vi "Disable.vi"(8 "error in (no error)":errorcluster, 11 "NhRegenGridSim in":refnum<class "NHRGridSim.lvclass">) -> (0 "error out":errorcluster, 3 "NhRegenGridSim out":refnum<class "NHRGridSim.lvclass">)   [LabVIEW 2018, in "AcPwrPlugins.lvlib" / "NHRGridSim.lvclass"]
doc: "This VI turns off the unit. Off is defined as the output relay being open."
uses:
  NHRGridSim.lvclass
  <instrlib>/NH Research 9400 Series/NH Research 9400 Series.lvlib
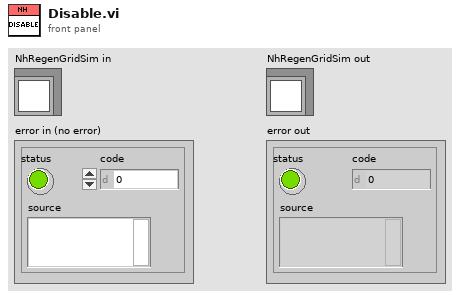
[diagram p1: front panel]
types:
  T1 = typedef "AcPwrPlugins.lvlib/NhRegenGridSim.lvclass/DeviceSettings.ctl" = cluster{"SlewRates":cluster{"Islew":dbl, "Vslew":dbl, "Pslew":dbl, "FreqSlew":dbl, "AngleABSlew":dbl, "AngleACSlew":dbl}, "Phases":cluster{"Pout (W)":dbl, "Iout (A)":dbl, "PhaseAngle":dbl, "Vout (V)":dbl, "Phase Name":string}[], "Measurement":cluster{"ApertureLength (s)":dbl, "NumberOfSamples":u32}, "Ranges":cluster{"Irange (A)":dbl, "Vrange (V)":dbl}, "Mode":enum8{"One 3-Phase AC", "One AC", "One DC", "Three AC", "Three DC", "One 2-Phase AC and One AC", "One 2-Phase AC and One DC", "Two AC", "One AC and One DC", "Two AC and One DC", "One AC and Two DC", "One DC and One AC", "Two DC"}, "PowerMax":u16, "TransformerRatio":dbl, "Waveshape":dbl[], "Handle":string, "FreqOut (Hz)":dbl, "Connected":bool, "Safety Limits":cluster{"Minimum Voltage (V)":dbl, "Minimum Voltage Time (s)":dbl, "Maximum Voltage (V)":dbl, "Maximum Voltage Time (s)":dbl, "Maximum Source Amps (A)":dbl, "Maximum Source Amps Time (s)":dbl, "Maximum Sink Amps (A)":dbl, "Maximum Sink Amps Time (s)":dbl, "Maximum Source Power (W)":dbl, "Maximum Source Power Time (s)":dbl, "Maximum Sink Power (W)":dbl, "Maximum Sink Power Time (s)":dbl, "Peak Voltage (V)":dbl, "Peak Voltage Enable":bool, "Peak Amps (A)":dbl, "Peak Amps Enable":bool}, "btnIdQuery":bool, "btnReset":bool}[]
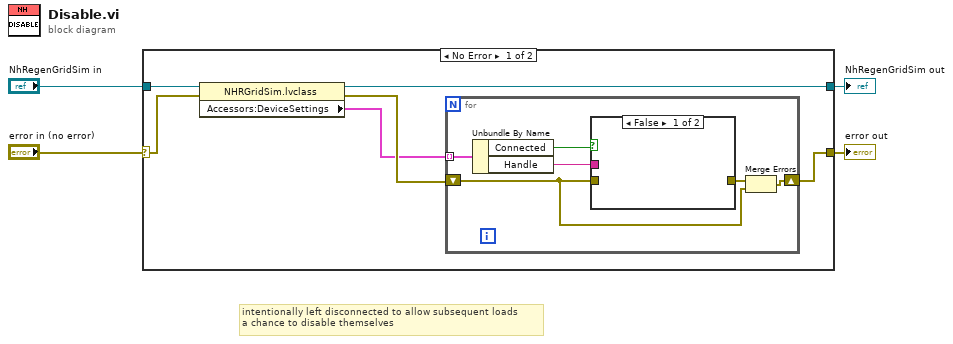
[diagram p0: block diagram]
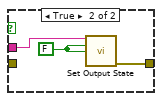
[diagram p2: hidden frame]
diagram:
  # "intentionally left disconnected to allow subsequent loads\na chance to disable themselves"
  n1 = case shown="No Error" "error in (no error)" {
    selector: "error in (no error)" -> [w9 w21]
    tunnel: [w6 w21] -> w4
    tunnel: [w8 w20] -> w3
    tunnel: "NhRegenGridSim in" -> [w10 w20]
    frame No Error {
      n2 = property class="NHRGridSim.lvclass"(reference=w10, error in=w9) -> (reference out=w8:refnum<class "NHRGridSim.lvclass">, error out=w7:errorcluster, "Accessors:DeviceSettings"=w5:T1)
      n3 = for {
        tunnel: w5 -> [w16] mode=indexing
        shift-right: [w12] -> w6
        shift-left: w7 -> [w11]
        n4 = Unbundle By Name(w16) -> ("Connected"=w14:bool, "Handle"=w15:string)
        n5 = case shown="False" w14 {
          tunnel: w11 -> [_ _]
          tunnel: [_ w19] -> w13
          tunnel: w15 -> [_ w17]
          frame False {
          }
          frame True {
            w18 = FALSE ("Output State (F: Disable)")
            n6 = call <instrlib>:"Set Output State.vi"("VISA resource name"=w17, "Output State (F: Disable)"=w18, "All (F: Disable)"=w18) -> ("error out"=w19:errorcluster)  [unwired: 11 in, 1 out]
          }
        }
        n7 = Merge Errors(w13, w11) -> (w12:errorcluster)
      }
    }
    frame Error {
    }
  }
  "error out" <- w4
  "NhRegenGridSim out" <- w3
